vi "MultiNPointAverager.vi"(8 "N point average":i32=20 min=0, 11 "Data_input":dbl) -> (3 "숫자형":dbl)   [LabVIEW 2024]
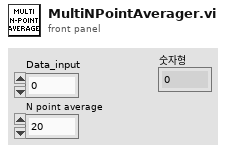
[diagram p1: front panel]
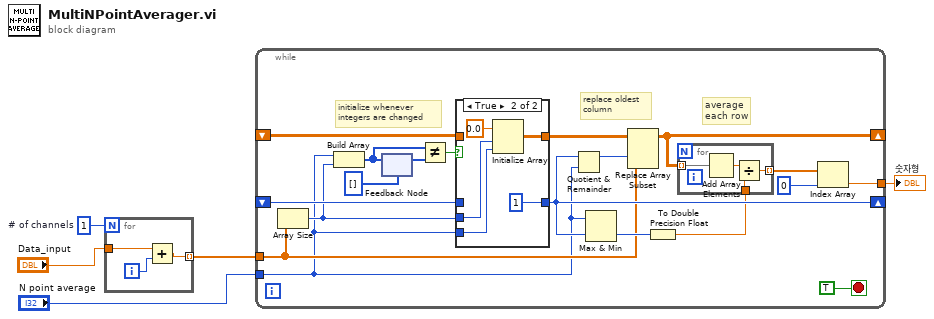
[diagram p0: block diagram]
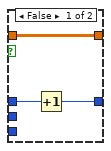
[diagram p2: hidden frame]
diagram:
  w5 = 1  # # of channels
  n1 = for {
    N: w5 -> [_]
    tunnel: "Data_input" -> [w7]
    tunnel: [w6] -> w3 mode=indexing
    i -> [w8]
    n2 = Add(x=w7, y=w8) -> (x+y=w6:dbl)
  }
  n3 = while {
    tunnel: w3 -> [w19]
    tunnel: "N point average" -> [w17]
    shift-right: [w24] -> _
    shift-left: _ -> [w22]
    shift-right: [w21] -> _
    shift-left: _ -> [w20]
    tunnel: [w9] -> w1
    stop <- TRUE stop-if-true
    # "average\neach row"
    # "initialize whenever\nintegers are changed"
    # "replace oldest\ncolumn"
    n4 = Array Size(array=w19) -> (size(s)=w18:i32)
    n5 = Build Array(w17, w18) -> (w15:i32[])
    n6 = feedback-in #1(w15) -> ()
    n7 = feedback #1(i32[] []) -> (w16:i32[])
    n8 = Not Equal?(x=w15, y=w16) -> (x != y?=w14:bool)
    n9 = case shown="True" w14 {
      tunnel: [w30 w33] -> w23
      tunnel: w22 -> [w30 _]
      tunnel: [w28 1] -> w21
      tunnel: w20 -> [w29 _]
      tunnel: w18 -> [_ w32]
      tunnel: w17 -> [_ w31]
      frame False {
        n10 = Increment(x=w29) -> (x+1=w28:i32)
      }
      frame True {
        n11 = Initialize Array(0.0 ("element"), w32, w31) -> (w33:dbl[][])
      }
    }
    n12 = Quotient & Remainder(x=w21, y=w17) -> (x-y*floor(x/y)=w27:i32)  [unwired: 1 out]
    n13 = Max & Min(x=w17, y=w21) -> (min(x,y)=w26:i32)  [unwired: 1 out]
    n14 = Replace Array Subset(array=w23, new element=w19, index (col)=w27) -> (w24:dbl[][])  [unwired: 1 in]
    n15 = To Double Precision Float(number=w26) -> (double precision float=w12:dbl)
    n16 = for {
      tunnel: w24 -> [w39] mode=indexing
      tunnel: w12 -> [w37]
      tunnel: [w36] -> w11 mode=indexing
      n17 = Add Array Elements(numeric array=w39) -> (sum=w38:dbl)
      n18 = Divide(x=w38, y=w37) -> (x/y=w36:dbl)
    }
    n19 = Index Array(array=w11, index=0) -> (element=w9:dbl)
  }
  "숫자형" <- w1
